vi "task2.4_4.vi"(11 "Frequency":dbl=10.0 format="%0.2p") -> (1 "A1 phase (deg)":dbl=264.9568956886852, 2 "A1 amplitude (db)":dbl=0.03331269437933233, 3 "A1 frequency (db) 2":dbl=0.03331269437933233)   [LabVIEW 2021]
doc: "This example demonstrates how to continuously re-generate analog output data from a buffer in your computer's memory.\n\nRefer to your device documentation for pinouts and hardware capabilities."
uses:
  <vilib>/DAQmx/write.llb/DAQmx Write (Analog Wfm 1Chan NSamp).vi
  <vilib>/DAQmx/write.llb/DAQmx Write (Digital Bool 1Line 1Point).vi
  <vilib>/DAQmx/read.llb/DAQmx Read (Analog 1D Wfm NChan NSamp).vi
  <vilib>/DAQmx/create/channels.llb/DAQmx Create Channel (AO-Voltage-Basic).vi
  <vilib>/DAQmx/configure/timing.llb/DAQmx Timing (Sample Clock).vi
  <vilib>/DAQmx/create/channels.llb/DAQmx Create Channel (AI-Voltage-Basic).vi
  <vilib>/DAQmx/configure/trigger.llb/DAQmx Start Trigger (Digital Edge).vi
  <vilib>/DAQmx/miscellaneous.llb/DAQmx Fill In Error Info.vi
  <vilib>/DAQmx/create/channels.llb/DAQmx Create Channel (DO-Digital Output).vi
  <vilib>/measure/matone.llb/Extract Single Tone Information N Chan.vi
  <vilib>/express/express analysis/Spectral/Block/exnSpectralBlock spectral measurements peak poly.vi
  <vilib>/express/express analysis/Spectral/Block/exnSpectralBlock spectral measurements peak array WFM.vi
  <vilib>/express/express analysis/Spectral/Block/exnSpectralBlock spectral measurements peak WFM.vi
  <vilib>/express/express analysis/Spectral/XNode/ExpressSpectralMeasurementsBlockNode.xnode
  <vilib>/measure/NI_MABase.lvlib
  <vilib>/measure/NI_MAPro.lvlib
panel:
  out "Output Freq":cluster{"f0":dbl, "df":dbl, "magnitude":dbl[]}(graph)
  out "Input Freq":cluster{"f0":dbl, "df":dbl, "magnitude":dbl[]}[](graph)
  in  "Amplitude":dbl=1.0 format="%0.2p"
  in  "Waveform Type":u16(ring) items=["Sine Wave", "Triangle Wave", "Square Wave", "Sawtooth Wave"]
  in  "Input Channel 2":tag="Dev3/ai1"
  in  "Number of samples":i32=1000
  out "Input Voltage":waveform(dbl)[](graph)=[{"t0"=timestamp(3702416907.610318 s since 1904-01-01), "dt"=9.999999999999999e-05, "Y"=array[1000 elements], "attributes"=variant("NI_ChannelName"=variant(string "Dev6/ai0"), "NI_UnitDescription"=variant(string "Volts"))}, {"t0"=timestamp(3702416907.610332 s since 1904-01-01), "dt"=9.999999999999999e-05, "Y"=array[1000 elements], "attributes"=variant("NI_ChannelName"=variant(string "Dev6/ai1"), "NI_UnitDescription"=variant(string "Volts"))}]
  in  "Input Channel 1":tag="Dev3/ai0"
  in  "Min Input Voltage":dbl=-10.0
  in  "Max Input Voltage":dbl=10.0
  in  "Output sample rate":dbl=10000.0 format="%0.2f"
  out "Output Voltage":waveform(dbl)(graph)={"t0"=timestamp(0 s since 1904-01-01), "dt"=0.0001, "Y"=array[1000 elements]}
  in  "Max Voltage":dbl=10.0
  in  "Min Voltage":dbl=-10.0
  in  "Output Channel":tag="Dev3/ao0"
  # "Output Channel Settings"
  # "Output voltage"
  # "Input voltage"
  # "Input Channel Settings"
  # "Waveform Settings"
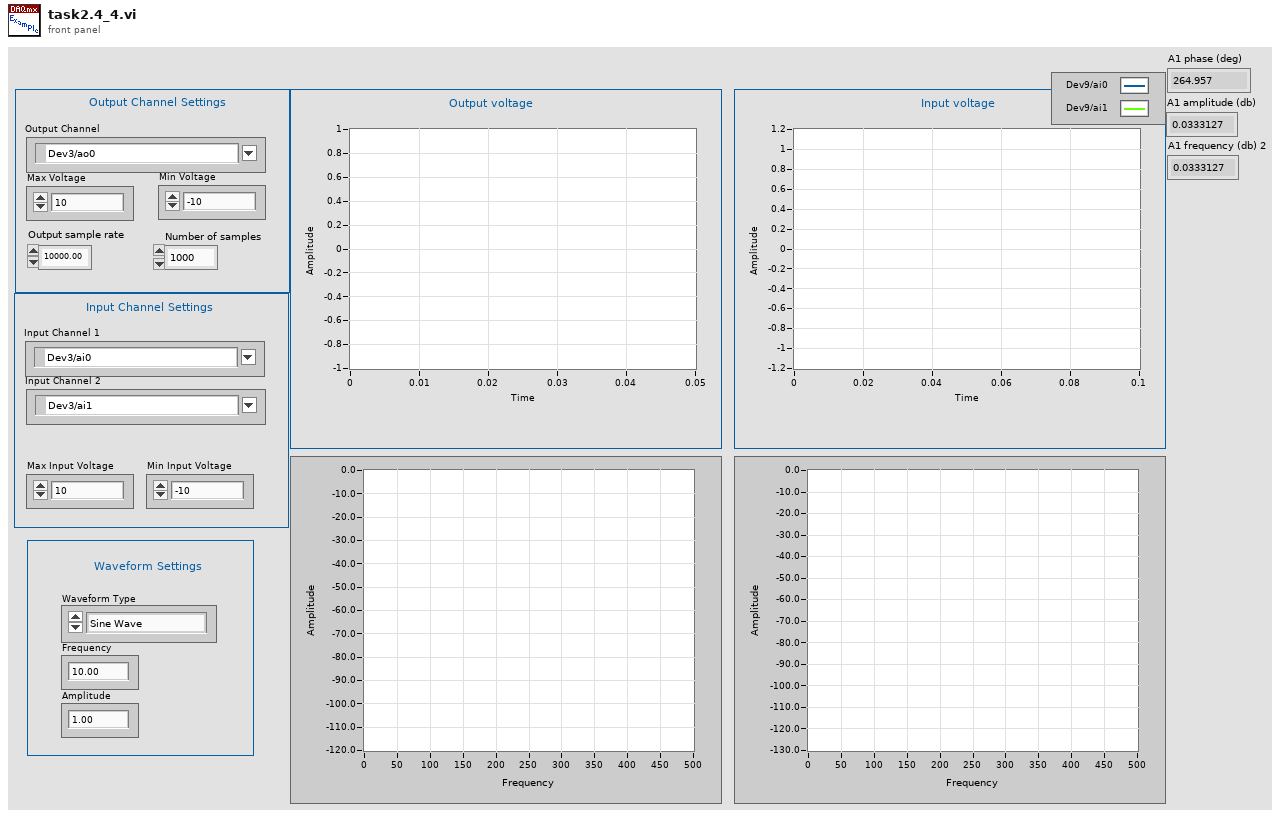
[diagram p1: front panel]
types:
  T1 = cluster{"Output sample rate":dbl, "Number of samples":i32}
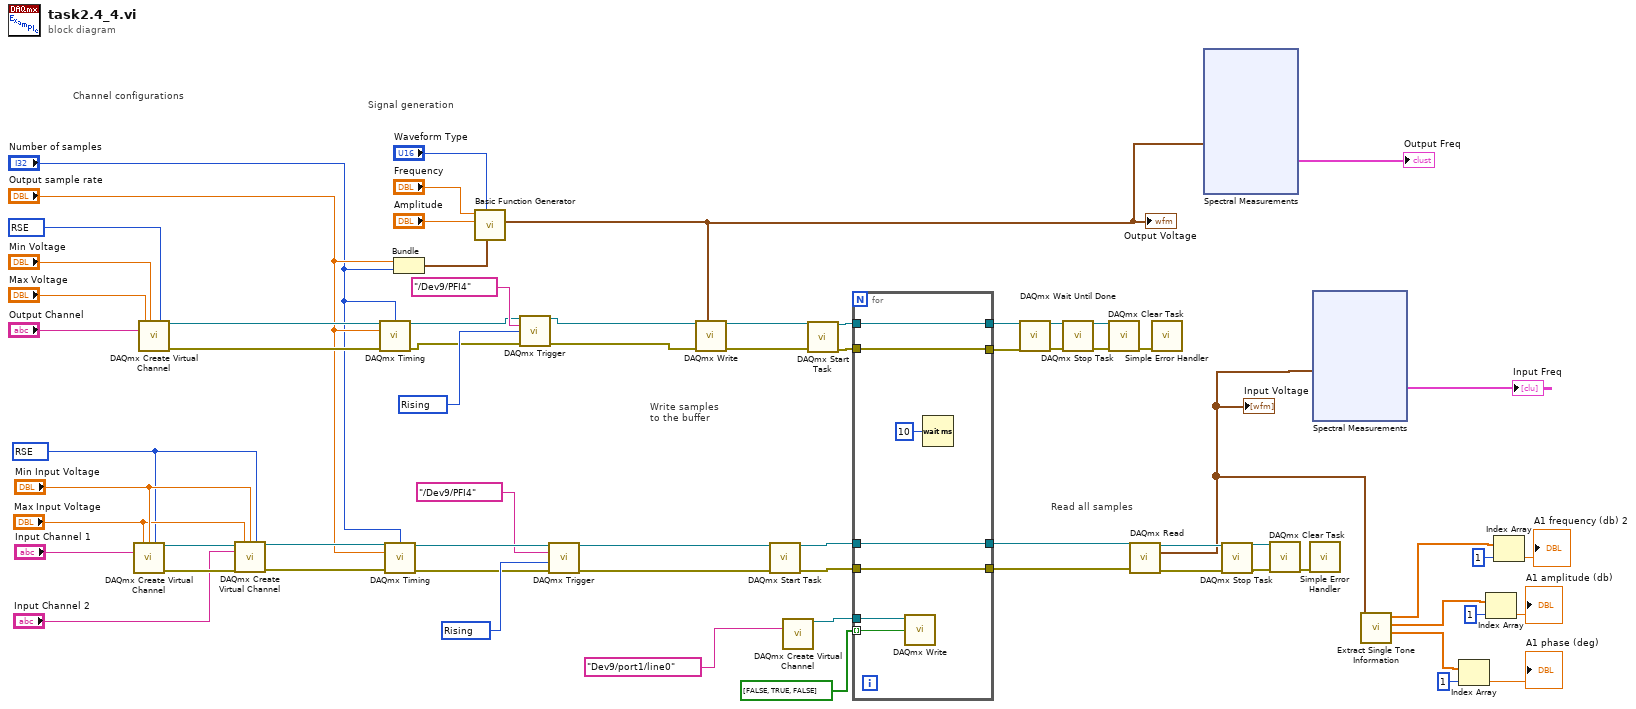
[diagram p0: block diagram]
diagram:
  w16 = 10280 items=["Rising"=10280, "Falling"=10171] ("edge")
  w20 = 10280 items=["Rising"=10280, "Falling"=10171] ("edge")
  w44 = 10083 items=["Default"=-1, "RSE"=10083, "NRSE"=10078, "Differential"=10106, "Pseudodifferential"=12529] ("input terminal configuration")
  w58 = 10083 items=["Default"=-1, "RSE"=10083, "NRSE"=10078, "Differential"=10106, "Pseudodifferential"=12529] ("input terminal configuration")
  # "Read all samples"
  # "Write samples\nto the buffer"
  # "Signal generation"
  # "Channel configurations"
  n1 = call-poly <vilib>:"DAQmx Create Virtual Channel.vi"("maximum value"="Max Input Voltage", "minimum value"="Min Input Voltage", "input terminal configuration"=w44, "physical channels"="Input Channel 1") -> ("task out"=w54:refnum<k21>, "error out"=w55:errorcluster)  [unwired: 10 in]
  n2 = call-poly <vilib>:"DAQmx Create Virtual Channel.vi"("maximum value"="Max Voltage", "minimum value"="Min Voltage", "output terminal configuration"=w58, "physical channels"="Output Channel") -> ("task out"=w62:refnum<k21>, "error out"=w63:errorcluster)  [unwired: 10 in]
  n3 = call-poly <vilib>:"DAQmx Create Virtual Channel.vi"("task in"=w54, "maximum value"="Max Input Voltage", "minimum value"="Min Input Voltage", "input terminal configuration"=w44, "physical channels"="Input Channel 2", "error in"=w55) -> ("task out"=w53:refnum<k21>, "error out"=w52:errorcluster)  [unwired: 8 in]
  n4 = call-poly <vilib>:"DAQmx Timing.vi"("task/channels in"=w62, "samples per channel"="Number of samples", "rate"="Output sample rate", "error in"=w63) -> ("task out"=w21:refnum<k21>, "error out"=w19:errorcluster)  [unwired: 10 in]
  n5 = call-poly <vilib>:"DAQmx Timing.vi"("task/channels in"=w53, "samples per channel"="Number of samples", "rate"="Output sample rate", "error in"=w52) -> ("task out"=w13:refnum<k21>, "error out"=w15:errorcluster)  [unwired: 10 in]
  n6 = Bundle "Bundle"("Output sample rate"="Output sample rate", "Number of samples"="Number of samples") -> (w43:T1)  [unwired: 1 in]
  n7 = call <vilib>:"Basic Function Generator.vi"("sampling info"=w43, "signal type"="Waveform Type", "amplitude"="Amplitude", "frequency"="Frequency") -> ("signal out"=w11:waveform(dbl))  [unwired: 5 in, 2 out]
  "Output Voltage" <- w11
  n8 = call-poly <vilib>:"DAQmx Trigger.vi"("task/channels in"=w21, "source"=tag "/Dev9/PFI4", "edge"=w20, "error in"=w19) -> ("task out"=w24:refnum<k21>, "error out"=w23:errorcluster)  [unwired: 10 in]
  n9 = call-poly <vilib>:"DAQmx Trigger.vi"("task/channels in"=w13, "source"=tag "/Dev9/PFI4", "edge"=w16, "error in"=w15) -> ("task out"=w18:refnum<k21>, "error out"=w17:errorcluster)  [unwired: 10 in]
  n10 = call-poly <vilib>:"DAQmx Write.vi"("task/channels in"=w24, "data"=w11, "error in"=w23) -> ("task out"=w26:refnum<k21>, "error out"=w25:errorcluster)  [unwired: 10 in, 1 out]
  n11 = call <vilib>:"DAQmx Start Task.vi"("task/channels in"=w18, "error in"=w17) -> ("task out"=w33:refnum<k21>, "error out"=w34:errorcluster)  [unwired: 12 in]
  n12 = call-poly <vilib>:"DAQmx Create Virtual Channel.vi"("lines"=tag "Dev9/port1/line0") -> ("task out"=w31:refnum<k21>)  [unwired: 13 in, 1 out]
  n13 = call <vilib>:"DAQmx Start Task.vi"("task/channels in"=w26, "error in"=w25) -> ("task out"=w35:refnum<k21>, "error out"=w36:errorcluster)  [unwired: 12 in]
  n14 = for {
    tunnel: bool[] [FALSE, TRUE, FALSE] -> [w75] mode=indexing
    tunnel: w34 -> [w71]
    tunnel: w33 -> [w72]
    tunnel: w36 -> [w73]
    tunnel: w35 -> [w74]
    tunnel: [w74] -> w30
    tunnel: [w73] -> w29
    tunnel: [w72] -> w28
    tunnel: [w71] -> w27
    tunnel: w31 -> [w70]
    n15 = call-poly <vilib>:"DAQmx Write.vi"("task/channels in"=w70, "data"=w75) -> ()  [unwired: 11 in, 3 out]
    n16 = Wait (ms)(milliseconds to wait=u32 10) -> ()  [unwired: 1 out]
  }
  n17 = call <vilib>:"DAQmx Wait Until Done.vi"("task/channels in"=w30, "error in"=w29) -> ("task out"=w40:refnum<k21>, "error out"=w39:errorcluster)  [unwired: 12 in]
  n18 = call <vilib>:"DAQmx Stop Task.vi"("task/channels in"=w40, "error in"=w39) -> ("task out"=w65:refnum<k21>, "error out"=w64:errorcluster)  [unwired: 12 in]
  n19 = call <vilib>:"DAQmx Clear Task.vi"("task in"=w65, "error in"=w64) -> ("error out"=w69:errorcluster)  [unwired: 13 in]
  n20 = call-poly <vilib>:"DAQmx Read.vi"("task/channels in"=w28, "error in"=w27) -> ("task out"=w56:refnum<k21>, "data"=w1:waveform(dbl)[], "error out"=w57:errorcluster)  [unwired: 11 in]
  "Input Voltage" <- w1
  n21 = call <vilib>:"Simple Error Handler.vi"("error in (no error)"=w69) -> ()  [unwired: 4 in, 5 out]
  n22 = xnode "Spectral Measurements"("Signals"=w11) -> ("FFT - (Peak)"=→"Output Freq":cluster{"f0":dbl, "df":dbl, "magnitude":dbl[]})  [unwired: 1 in, 2 out]
  n23 = call <vilib>:"DAQmx Stop Task.vi"("task/channels in"=w56, "error in"=w57) -> ("task out"=w60:refnum<k21>, "error out"=w61:errorcluster)  [unwired: 12 in]
  n24 = call <vilib>:"DAQmx Clear Task.vi"("task in"=w60, "error in"=w61) -> ("error out"=w59:errorcluster)  [unwired: 13 in]
  n25 = call <vilib>:"Simple Error Handler.vi"("error in (no error)"=w59) -> ()  [unwired: 4 in, 5 out]
  n26 = xnode "Spectral Measurements"("Signals"=w1) -> ("FFT - (Peak)"=→"Input Freq":cluster{"f0":dbl, "df":dbl, "magnitude":dbl[]}[])  [unwired: 1 in, 2 out]
  n27 = call-poly <vilib>:"Extract Single Tone Information.vi"("time signals in"=w1) -> ("detected phases (deg)"=w7:dbl[], "detected amplitudes"=w9:dbl[], "detected frequencies"=w2:dbl[])  [unwired: 5 in, 3 out]
  n28 = Index Array(array=w7, index=1) -> (element=→"A1 phase (deg)":dbl)
  n29 = Index Array(array=w9, index=1) -> (element=→"A1 amplitude (db)":dbl)
  n30 = Index Array(array=w2, index=1) -> (element=→"A1 frequency (db) 2":dbl)
